vi "RunOperation.vi"(10 "Inputs":string[](array[string]), 11 "ExecuteMultipleBuildSpecs in":refnum<class "ExecuteMultipleBuildSpecs.lvclass">) -> (1 "Output/Failure message":string, 2 "CLI Process Return Code":i32, 3 "ExecuteMultipleBuildSpecs out":refnum<class "ExecuteMultipleBuildSpecs.lvclass">)   [LabVIEW 2014, in "ExecuteMultipleBuildSpecs.lvclass"]
doc: "Entry point for LabVIEWCLI."
uses:
  ExecuteMultipleBuildSpecs.lvclass
  ExecuteMultipleBuildSpecs.lvclass/ExecuteMultipleBuildSpecs.ctl
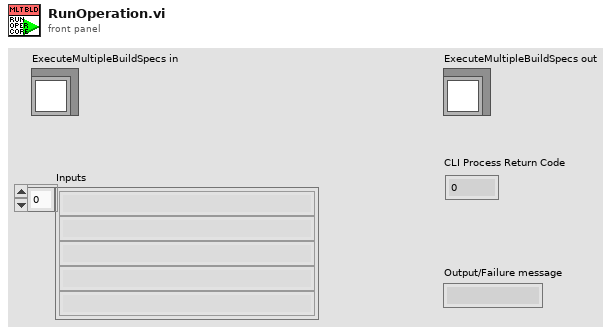
[diagram p1: front panel]
types:
  T1 = typedef "ExecuteMultipleBuildSpecs.lvclass/SpecInformation.ctl" = cluster{"Target":string, "Build Spec":string}
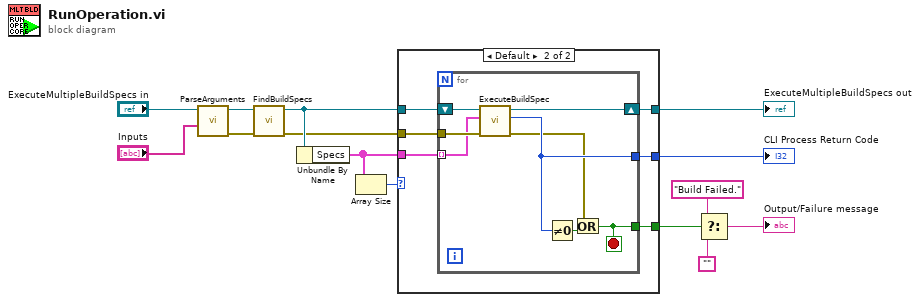
[diagram p0: block diagram]
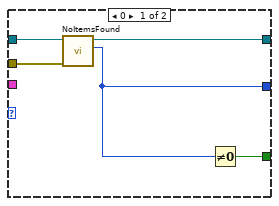
[diagram p2: hidden frame]
diagram:
  n1 = call "ParseArguments.vi"("Inputs"="Inputs", "ExecuteMultipleBuildSpecs in"="ExecuteMultipleBuildSpecs in") -> ("error out"=w12:errorcluster, "ExecuteMultipleBuildSpecs out"=w13:refnum<class "ExecuteMultipleBuildSpecs.lvclass">)  [unwired: 8 in]
  n2 = call "FindBuildSpecs.vi"("error in (no error)"=w12, "ExecuteMultipleBuildSpecs in"=w13) -> ("error out"=w9:errorcluster, "ExecuteMultipleBuildSpecs out"=w11:refnum<class "ExecuteMultipleBuildSpecs.lvclass">)  [unwired: 8 in]
  n3 = Unbundle By Name(w11) -> ("Specs"=w3:T1[])
  n4 = Array Size(array=w3) -> (size(s)=w2:i32)
  n5 = case shown="Default" w2 {
    tunnel: w11 -> [w17 w25]
    tunnel: [w16 w24] -> w10
    tunnel: w9 -> [w18 w23]
    tunnel: [w15 w22] -> w8
    tunnel: w3 -> [_ w21]
    tunnel: [w19 w20] -> w7
    frame 0 {
      n6 = call "NoItemsFound.vi"("error in (no error)"=w18, "ExecuteMultipleBuildSpecs in"=w17) -> ("CLI Process Return Code"=w15:i32, "ExecuteMultipleBuildSpecs out"=w16:refnum<class "ExecuteMultipleBuildSpecs.lvclass">)  [unwired: 8 in]
      n7 = Not Equal To 0?(x=w15) -> (x != 0?=w19:bool)
    }
    frame Default {
      n8 = for {
        shift-right: [w32] -> w24
        shift-left: w25 -> [w33]
        tunnel: w21 -> [w30] mode=indexing
        tunnel: [w29] -> w22
        tunnel: [w26] -> w20
        tunnel: w23 -> [w31]
        stop <- w26 stop-if-true
        n9 = call "ExecuteBuildSpec.vi"("error in (no error)"=w31, "Spec Info"=w30, "ExecuteMultipleBuildSpecs in"=w33) -> ("error out"=w28:errorcluster, "CLI Process Return Code"=w29:i32, "ExecuteMultipleBuildSpecs out"=w32:refnum<class "ExecuteMultipleBuildSpecs.lvclass">)  [unwired: 5 in, 1 out]
        n10 = Not Equal To 0?(x=w29) -> (x != 0?=w27:bool)
        n11 = Or(x=w28, y=w27) -> (x .or. y?=w26:bool)
      }
    }
  }
  "ExecuteMultipleBuildSpecs out" <- w10
  "CLI Process Return Code" <- w8
  n12 = Select(t="Build Failed.", s=w7, f="") -> (s? t:f=→"Output/Failure message":string)
